vi "last_density_query.vi"(8 "error in (no error)":errorcluster, 11 "Small?":bool) -> (0 "error out":errorcluster, 3 "Density":dbl)   [LabVIEW 2013]
uses:
  <vilib>/addons/database/_DB Variant To Data/Database Variant To Data.xnode
panel:
  out "SQL Query":string
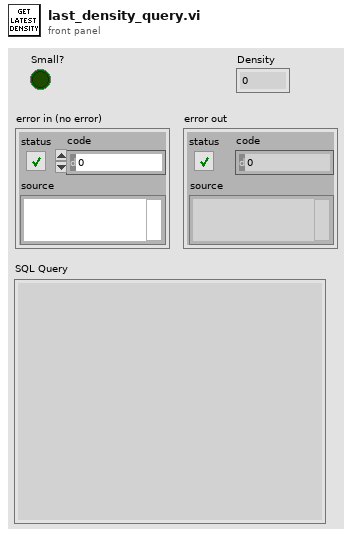
[diagram p1: front panel]
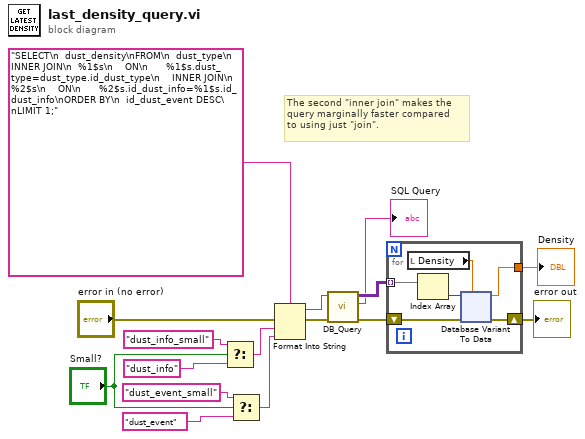
[diagram p0: block diagram]
diagram:
  # "The second \"inner join\" makes the\nquery marginally faster compared\nto using just \"join\"."
  n1 = Select(t="dust_info_small", s="Small?", f="dust_info") -> (s? t:f=w10:string)
  n2 = Select(t="dust_event_small", s="Small?", f="dust_event") -> (s? t:f=w9:string)
  n3 = Format Into String(format string="SELECT\n  dust_density\nFROM\n  dust_type\n    INNER JOIN\n  %1$s\n    ON\n      %1$s.dust_type=dust_type.id_dust_type\n    INNER JOIN\n  %2$s\n    ON\n      %2$s.id_dust_info=%1$s.id_dust_info\nORDER BY\n  id_dust_event DESC\nLIMIT 1;", error in="error in (no error)", w10, w9) -> (resulting string=w2:string, error out=w5:errorcluster)  [unwired: 1 in]
  n4 = call "DB_Query.vi"("error in (no error)"=w5, "Parameterized Query"=w2) -> ("error out"=w4:errorcluster, "Query in Standard Format"=→"SQL Query":string, "Results"=w3:variant[][])  [unwired: 7 in]
  n5 = for {
    tunnel: [w21] -> w7
    shift-right: [w22] -> w16
    shift-left: w4 -> [w17]
    tunnel: w3 -> [w18] mode=indexing
    n6 = local read "Density"() -> (w19:dbl)
    n7 = Index Array(array=w18) -> (element=w20:variant)  [unwired: 1 in]
    n8 = xnode "Database Variant To Data"("database variant"=w20, "error in (no error)"=w17, "type"=w19) -> ("data"=w21:dbl, "error out"=w22:errorcluster)
  }
  "error out" <- w16
  "Density" <- w7
